vi "set motor settings.vi"(8 "error in (no error)":errorcluster, 10 "motor_settings":T1, 11 "id":i32) -> (0 "error out":errorcluster, 3 "function return":i32)   [LabVIEW 2012, in "libximc.lvlib"]
doc: "result_t XIMC_API set_motor_settings (device_t id, const motor_settings_t* motor_settings);"
uses:
  libximc.lvlib
  libximc.dll
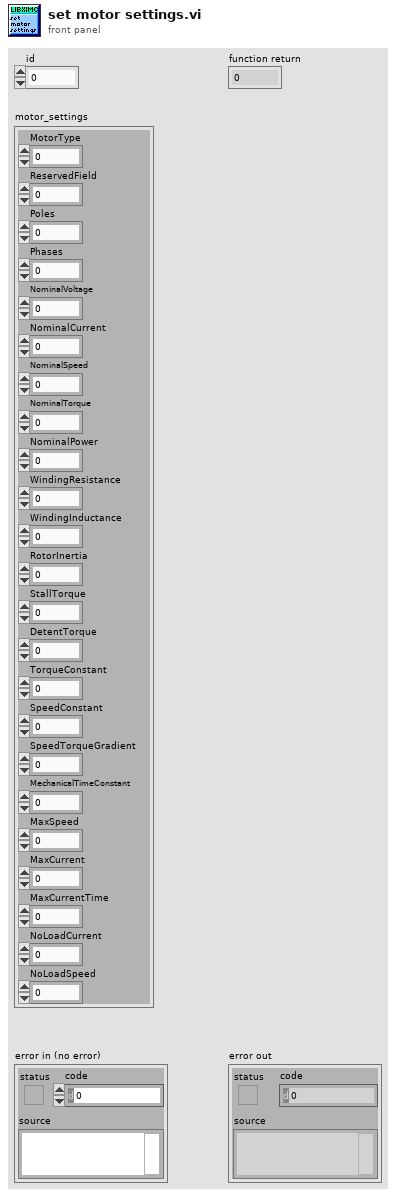
[diagram p1: front panel]
types:
  T1 = cluster{"MotorType":u32, "ReservedField":u32, "Poles":u32, "Phases":u32, "NominalVoltage":sgl, "NominalCurrent":sgl, "NominalSpeed":sgl, "NominalTorque":sgl, "NominalPower":sgl, "WindingResistance":sgl, "WindingInductance":sgl, "RotorInertia":sgl, "StallTorque":sgl, "DetentTorque":sgl, "TorqueConstant":sgl, "SpeedConstant":sgl, "SpeedTorqueGradient":sgl, "MechanicalTimeConstant":sgl, "MaxSpeed":sgl, "MaxCurrent":sgl, "MaxCurrentTime":sgl, "NoLoadCurrent":sgl, "NoLoadSpeed":sgl}
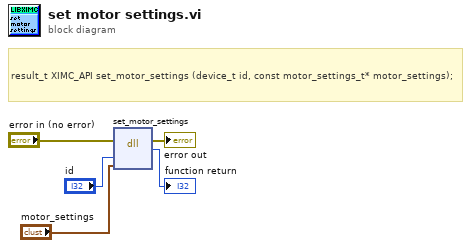
[diagram p0: block diagram]
diagram:
  # "result_t XIMC_API set_motor_settings (device_t id, const motor_settings_t* motor_settings);"
  n1 = dll-call lib="C:/Users/user/Desktop/labview-2.9.11-gen/libximc.*" fn="set_motor_settings"(error in="error in (no error)", "id"="id", "motor_settings"="motor_settings") -> (error out=→"error out":errorcluster, →"function return":i32)  [unwired: 4 in, 1 out]
